vi "PCAN_READ.vi"(7 "pathCAN_DLL":path, 8 "error in (no error)":errorcluster) -> (0 "error out":errorcluster, 2 "TPCANMsg":T2 {"ID" format="%x"; "MSGTYPE" items=["STATUS"=128, "EXTENDED"=2, "RTR"=1, "DATA MSG"=0]; "aDATA" format="%x"}, 3 "error":T1 items=["CAN_ERR_OK"=0, "CAN_ERR_XMTFULL"=1, "CAN_ERR_OVERRUN"=2, "CAN_ERR_BUSLIGHT"=4, "CAN_ERR_BUSHEAVY"=8, "CAN_ERR_BUSOFF"=16, "CAN_ERR_QRCVEMPTY"=32, "CAN_ERR_QOVERRUN"=64, "CAN_ERR_QXMTFULL"=128, "CAN_ERR_REGTEST"=256, "CAN_ERR_NOVXD"=512, "CAN_ERR_HWINUSE"=1024, "CAN_ERR_NETINUSE"=2048, "CAN_ERR_ILLHW"=5120, "CAN_ERR_ILLNET"=6144, "CAN_ERR_ILLCLINET"=7168, "CAN_ERR_RESOURCE"=8192, "CAN_ERR_ILLPARAMTYPE"=16384, "CAN_ERR_ILLPARAMVAL"=32768, "CAN_ERR_UNKNOWN"=65536])   [LabVIEW 2023, in "pCANLib.lvlib"]
doc: "///////////////////////////////////////////////////////////////////////////////\n// CAN_Read()\n// gibt die naechste Message oder den naechsten Fehler aus dem\n// RCV-Queue des Clients zurueck.\n//\n// CAN_Read() gibt die nächste Message oder den nächsten Fehler aus dem RCV-Queue des Clients zurück. Message wird\n// nach 'msgbuff' geschrieben. ACHTUNG der MSG_Type gibt an ob es sich um eine 11Bit, 29Bit, RTR oder Status\n// Nachricht handelt. IMMER abfragen !. \n// \n// Ist die gelesene CAN Nachricht keine normale Nachricht sondern eine Statusmeldung so ist der Rueckgabewert \n// der CAN_Read() Funktion weiterhin CAN_ERR_OK, jedoch ist in TPCAN_MSG Struktur der MSGTYPE = MSGTYPE_STATUS.\n// \n// Identifier und Laegencode einer solchen Statusnachricht duerfen nicht ausgewertet werden (undefinierte Werte).\n// Die eigentliche Information ueber den Fehler lassen sich nun aus den ersten 4 Datenbytes der Nachricht \n// herauslesen:\n// \n// Data0 Data1 Data2 Data3 Fehlertyp\n// 0x00 0x00 0x00 0x02 == CAN_ERR_OVERRUN 0x0002 // CAN-Controller wurde zu spaet gelesen\n// 0x00 0x00 0x00 0x04 == CAN_ERR_BUSLIGHT 0x0004 // Busfehler: ein Errorcounter erreichte Limit (96)\n// 0x00 0x00 0x00 0x08 == CAN_ERR_BUSHEAVY 0x0008 // Busfehler: ein Errorcounter erreichte Limit (128)\n// \n// 0x00 0x00 0x00 0x10 == CAN_ERR_BUSOFF 0x0010 // Busfehler: CAN_Controller ging 'Bus-Off'\n// \n// Beim Empfangen einer BUSOFF Statusnachricht ist der CAN-Controller mit CAN_Init() neu zu initialisieren,\n// da sonst keine Nachrichtem mehr gesendet werden koennen!\n// \n// \n// Message wird nach 'msgbuff' geschrieben.\n// moegliche Fehler: NOVXD QRCVEMPTY\n//\n\nDWORD __stdcall CAN_Read(TPCANMsg* pMsgBuff );"
uses:
  pCANLib.lvlib
  PCAN_ERROR.ctl
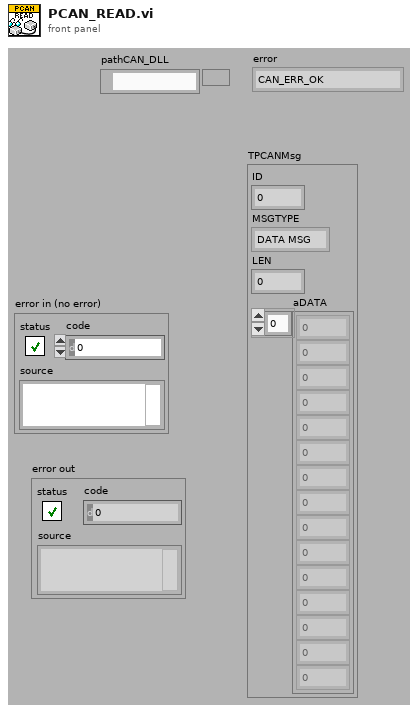
[diagram p1: front panel]
types:
  T1 = typedef "pCANLib.lvlib/PCAN_ERROR.ctl" = i32
  T2 = cluster{"ID":u32, "MSGTYPE":u8, "LEN":u8, "aDATA":u8[]}
  T3 = enum16{"big-endian, network order", "native, host order", "little-endian"}
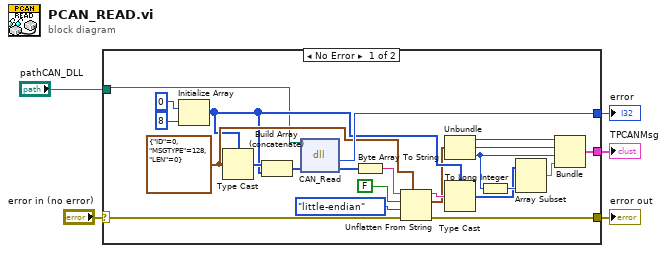
[diagram p0: block diagram]
diagram:
  n1 = case shown="No Error" "error in (no error)" {
    selector: "error in (no error)" -> [w19 w29]
    tunnel: [w28 _] -> w2
    tunnel: [w26 w29] -> w4
    tunnel: [w14 _] -> w3
    tunnel: "pathCAN_DLL" -> [w6 _]
    frame No Error {
      w20 = cluster{"ID":u32, "MSGTYPE":u8, "LEN":u8} {"ID"=0, "MSGTYPE"=128, "LEN"=0} ("TPCANMsg")
      n2 = Initialize Array(u8 0 ("DATA"), 8 ("dimension size")) -> (w16:u8[])
      n3 = Type Cast(type=w16, x=w20) -> (*(type *) &x=w17:u8[])
      n4 = Build Array (concatenate)(w17, w16) -> (w15:u8[])
      n5 = dll-call lib="D:/PCAN/PCAN/PCAN Driver/PCAN_Driver/PCAN_USB.DLL" fn="CAN_Read"(path in=w6, "pMsgBuff"=w15) -> ("return type"=w28:i32, "pMsgBuff"=w25:u8[])  [unwired: 2 in, 2 out]
      n6 = Byte Array To String(unsigned byte array=w25) -> (string=w27:string)
      n7 = Unflatten From String(type=w20, binary string=w27, data includes array or string size? (T)=FALSE ("prepend array or string size? (T)"), byte order (0:big-endian, network order)=T3."little-endian", error in (no error)=w19) -> (rest of the binary string=w18:string, value=w13:cluster{"ID":u32, "MSGTYPE":u8, "LEN":u8}, error out=w26:errorcluster)
      n8 = Unbundle(w13) -> ("ID"=w11:u32, "MSGTYPE"=w12:u8, "LEN"=w7:u8)
      n9 = Type Cast(type=w16, x=w18) -> (*(type *) &x=w9:u8[])
      n10 = To Long Integer(number=w7) -> (32bit integer=w10:i32)
      n11 = Array Subset(array=w9, length=w10) -> (w8:u8[])  [unwired: 1 in]
      n12 = Bundle("ID"=w11, "MSGTYPE"=w12, "LEN"=w7, w8) -> (w14:cluster{"ID":u32, "MSGTYPE":u8, "LEN":u8, u8[]})  [unwired: 1 out]
    }
    frame Error {
    }
  }
  "error out" <- w4
  "TPCANMsg" <- w3
  "error" <- w2
